vi "read N samples N channels.vi"(8 "error in (no error)":errorcluster, 11 "DAQ  in":refnum<class "DAQ .lvclass">) -> (0 "error out":errorcluster, 2 "data 2":waveform(dbl)[](array[waveform]), 3 "DAQ  out":refnum<class "DAQ .lvclass">)   [LabVIEW 2017, in "Hardware.lvlib" / "DAQ .lvclass"]
uses:
  DAQ .lvclass
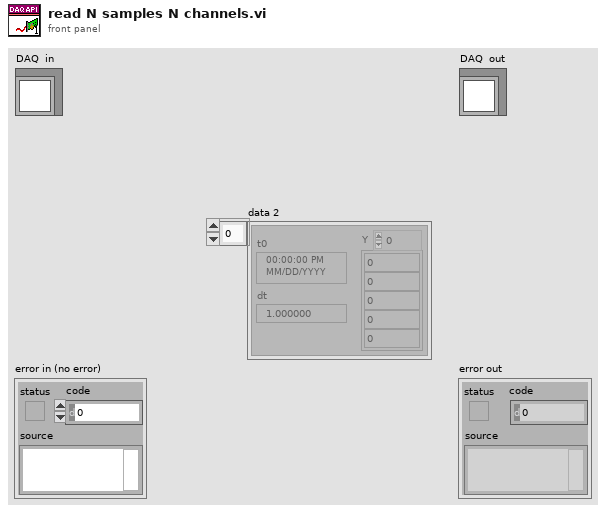
[diagram p1: front panel]
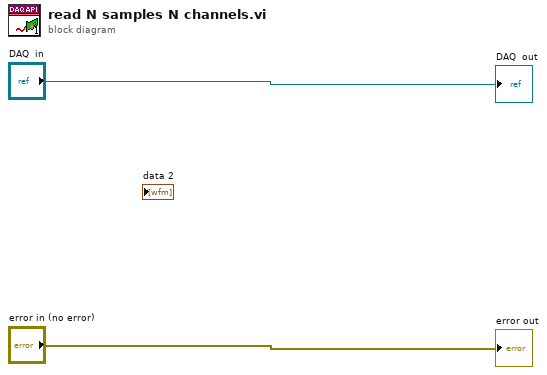
[diagram p0: block diagram]
diagram:
  "error out" <- "error in (no error)"
  "DAQ  out" <- "DAQ  in"
